vi "AlliGator Action Loop.vi"(8 "Error In":errorcluster, 10 "AlliGator Ctrl Refnums":T1, 11 "AlliGator Refnum":refnum<vi>) -> (0 "Error Out":errorcluster)   [LabVIEW 2021, in "AlliGator Action Engine.lvlib"]
doc: "AlliGator action dispatcher.\nEach action array is handled as a package, each action in the array being sent to the appropriate category (Files, Image, Phasor Graph, etc.)."
uses:
  AlliGator Action Engine.lvlib
  AlliGator Ctrl Refnums.ctl
  AlliGator Other Ctrl Refnums.ctl
  AlliGator State Indicator.ctl
  AlliGator Main Window Tabs.ctl
  AlliGator Phasor Plot Ctrl Refnums.ctl
  AlliGator Phasor Graph Ctrl Refnums.ctl
  Phasor/Phasor Calibration Type.ctl
  AlliGator Dataset Ctrl Refnums.ctl
  AlliGator Displayed Image.ctl
  AlliGator Registered Events Ctrl Refnums.ctl
  AlliGator Image Histogram Control Refnums.ctl
  Histograms/Linear Histogram Options.ctl
  Histograms/Histogram Bin Option.ctl
  Histograms/Histogram Bin Position.ctl
  AlliGator Decay Fit Map Control Refnums.ctl
  Fits/IRF(X)PSED/Decay Fit Parameters & Derived Quantities List.ctl
  AlliGator Internal Variables v2.ctl
  <vilib>/vision/Image Controls.llb/IMAQ Image.ctl
  AlliGator Gate Image Set.ctl
  AlliGator FLI Dataset Type.ctl
  AlliGator Data Series Type.ctl
  AlliGator Dataset Channel.ctl
  AlliGator Gate Arithmetic.ctl
  Image/Named ROI Description.ctl
  AlliGator Decay Metadata v3.ctl
  AlliGator Decay Background Subtraction Info.ctl
  AlliGator Baseline Subtraction Method.ctl
  Graphs/XY Graph/XY Graph Plot Shift Parameters.ctl
  Graphs/XY Graph/XY Graph Plot Shift Method.ctl
  AlliGator Decay Extrapolation Parameters.ctl
  Phasor/Calibration Phasor (m, phi).ctl
  Phasor/Phasor Reference Series.ctl
  Phasor/Phasor Calibration Map v2.ctl
  Phasor/Phasor (g, s).ctl
  AlliGator Raw Phasor Plot Data v4.ctl
  Phasor/Phasor Standard Deviation Options.ctl
  AlliGator Phasor Multi-Harmonic Data.ctl
  Phasor/Phasor Harmonic Data.ctl
  AlliGator Decay Fit Options & Parameters v2.ctl
  Fits/IRF(X)PSED/Decay Fit Options v2.ctl
  Fits/Decay Convolution/Decay Model.ctl
  Fits/Residual Type.ctl
  Fits/IRF(X)PSED/Fit Weights Type.ctl
  Fits/Non-linear Fitting Method v2.ctl
  Fits/Fit Calculation Method.ctl
  Fits/Non-linear Fitting Algorithm.ctl
  AlliGator Decay Fit Parameter Constraints 2.ctl
  Fits/IRF(X)PSED/Decay Fit Parameters In List.ctl
  Fits/IRF(X)PSED/MLE Baseline Offset Type.ctl
  AlliGator Decay Preprocessing Parameters.ctl
  AlliGator Parameter Maps Data.ctl
  AlliGator Q Event.ctl
  AlliGator Settings List.ctl
  Graphs/XY Graph/XY Graph Selected Plot Info.ctl
  Graphs/XY Graph/XY Graph Refnum.ctl
  <vilib>/Utility/miscctls.llb/LVPoint32TypeDef.ctl
  Graphs/XY Graph/XY Graph Mouse Click Event Data.ctl
  AlliGator Debug Action List.ctl
  Alligator Elements Order in Action Stack.ctl
  bb653f8f-7323-4417-bc10-ef5a2241dee5.vi
  AlliGator Globals.vi
  Variant/Variant to Data/Variant to Boolean.vi
  AlliGator Add Action Array to Stack.vi
  Error/Error.lvlib
  Utilities/Utilities.lvlib
  AlliGator GUI.lvlib
  Notebook/Notebook.lvlib
  AlliGator Globals, Variables & Constants.lvlib
  AlliGator Settings.lvlib
  Graphs/XY Graph/XY Graph Add-Ons.lvlib
  Variant/Variant to Data/Variant to Data.lvlib
  AlliGator Debug.lvlib
  Phasor/Phasor.lvlib
  Image/Image.lvlib
  AlliGator Decay Preprocessing.lvlib
  AlliGator Phasor Graph.lvlib
  AlliGator Files.lvlib
  AlliGator Internal Variables.lvlib
  AlliGator Phasor Plot.lvlib
  AlliGator Source Image.lvlib
  Fits/Fits.lvlib
  AlliGator Decay Fit.lvlib
  AlliGator Decay Fit Parameter Map.lvlib
  AlliGator Python Plugins.lvlib
  AlliGator Dual-Channel Datasets.lvlib
  Histograms/Histogram Window.lvlib
panel:
  # "Drop the content of this VI on AlliGator's diagram\nIn AlliGator, replace the subVI template by a new version"
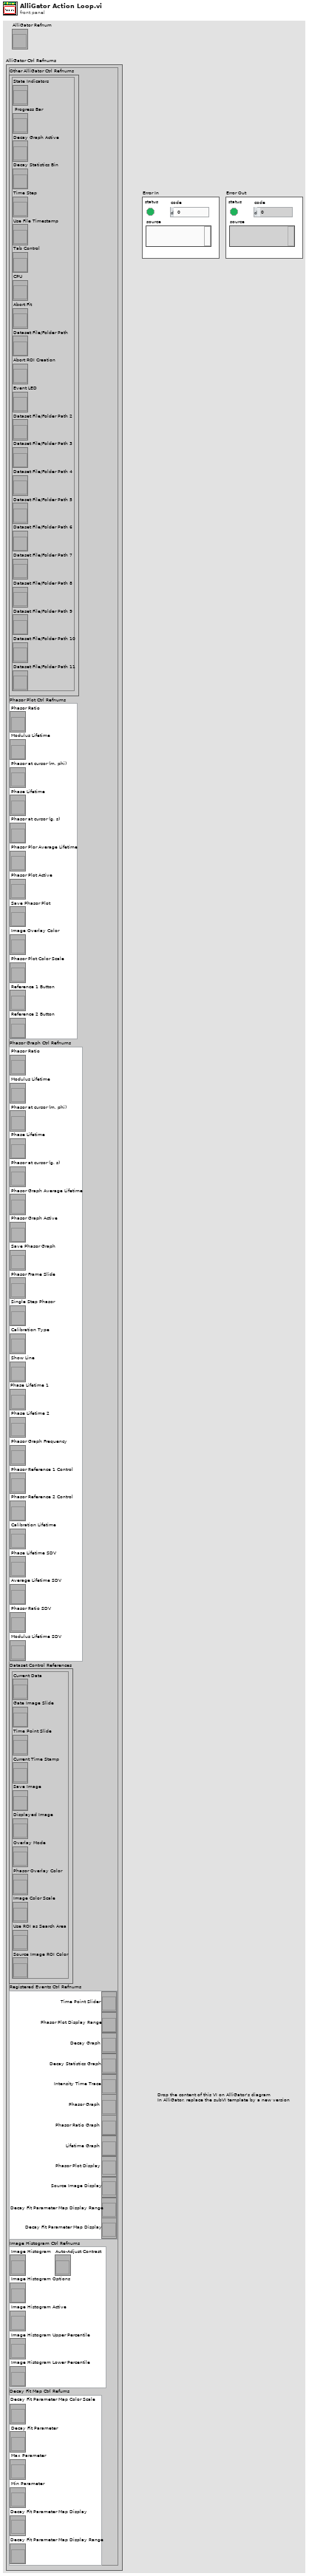
[diagram p1: front panel]
types:
  T1 = typedef "AlliGator GUI.lvlib/AlliGator Ctrl Refnums.ctl" = cluster{"Other AlliGator Ctrl Refnums":T2, "Phasor Plot Ctrl Refnums":T3, "Phasor Graph Ctrl Refnums":T4, "Dataset Control References":T5, "Registered Events Ctrl Refnums":T6, "Image Histogram Ctrl Refnums":T7, "Decay Fit Map Ctrl Refums":T8}
  T2 = typedef "AlliGator GUI.lvlib/AlliGator Other Ctrl Refnums.ctl" = cluster{"State Indicators":refnum<vi>, " Progress Bar":refnum<vi>, "Decay Graph Active":refnum<vi>, "Decay Statistics Bin":refnum<vi>, "Time Step":refnum<vi>, "Use File Timestamp":refnum<vi>, "Tab Control":refnum<vi>, "CPU":refnum<vi>, "Abort Fit":refnum<vi>, "Dataset File/Folder Path":refnum<vi>, "Abort ROI Creation":refnum<vi>, "Event LED":refnum<vi>, "Dataset File/Folder Path 2":refnum<vi>, "Dataset File/Folder Path 3":refnum<vi>, "Dataset File/Folder Path 4":refnum<vi>, "Dataset File/Folder Path 5":refnum<vi>, "Dataset File/Folder Path 6":refnum<vi>, "Dataset File/Folder Path 7":refnum<vi>, "Dataset File/Folder Path 8":refnum<vi>, "Dataset File/Folder Path 9":refnum<vi>, "Dataset File/Folder Path 10":refnum<vi>, "Dataset File/Folder Path 11":refnum<vi>}
  T3 = typedef "AlliGator GUI.lvlib/AlliGator Phasor Plot Ctrl Refnums.ctl" = cluster{"Phasor Ratio":refnum<vi>, "Modulus Lifetime":refnum<vi>, "Phasor at cursor (m, phi)":refnum<vi>, "Phase Lifetime":refnum<vi>, "Phasor at cursor (g, s)":refnum<vi>, "Phasor Plor Average Lifetime":refnum<vi>, "Phasor Plot Active":refnum<vi>, "Save Phasor Plot":refnum<vi>, "Image Overlay Color":refnum<vi>, "Phasor Plot Color Scale":refnum<vi>, "Reference 1 Button":refnum<vi>, "Reference 2 Button":refnum<vi>}
  T4 = typedef "AlliGator GUI.lvlib/AlliGator Phasor Graph Ctrl Refnums.ctl" = cluster{"Phasor Ratio":refnum<vi>, "Modulus Lifetime":refnum<vi>, "Phasor at cursor (m, phi)":refnum<vi>, "Phase Lifetime":refnum<vi>, "Phasor at cursor (g, s)":refnum<vi>, "Phasor Graph Average Lifetime":refnum<vi>, "Phasor Graph Active":refnum<vi>, "Save Phasor Graph":refnum<vi>, "Phasor Frame Slide":refnum<vi>, "Single Step Phasor":refnum<vi>, "Calibration Type":refnum<vi>, "Show Line":refnum<vi>, "Phase Lifetime 1":refnum<vi>, "Phase Lifetime 2":refnum<vi>, "Phasor Graph Frequency":refnum<vi>, "Phasor Reference 1 Control":refnum<vi>, "Phasor Reference 2 Control":refnum<vi>, "Calibration Lifetime":refnum<vi>, "Phase Lifetime SDV":refnum<vi>, "Average Lifetime SDV":refnum<vi>, "Phasor Ratio SDV":refnum<vi>, "Modulus Lifetime SDV":refnum<vi>}
  T5 = typedef "AlliGator GUI.lvlib/AlliGator Dataset Ctrl Refnums.ctl" = cluster{"Current Data":refnum<vi>, "Gate Image Slide":refnum<vi>, "Time Point Slide":refnum<vi>, "Current Time Stamp":refnum<vi>, "Save Image":refnum<vi>, "Displayed Image":refnum<vi>, "Overlay Mode":refnum<vi>, "Phasor Overlay Color":refnum<vi>, "Image Color Scale":refnum<vi>, "Use ROI as Search Area":refnum<vi>, "Source Image ROI Color":refnum<vi>}
  T6 = typedef "AlliGator GUI.lvlib/AlliGator Registered Events Ctrl Refnums.ctl" = cluster{"Time Point Slider":refnum<vi>, "Phasor Plot Display Range":refnum<vi>, "Decay Graph":refnum<vi>, "Decay Statistics Graph":refnum<vi>, "Intensity Time Trace":refnum<vi>, "Phasor Graph":refnum<vi>, "Phasor Ratio Graph":refnum<vi>, "Lifetime Graph":refnum<vi>, "Phasor Plot Display":refnum<vi>, "Source Image Display":refnum<vi>, "Decay Fit Parameter Map Display Range":refnum<vi>, "Decay Fit Parameter Map Display":refnum<vi>}
  T7 = typedef "AlliGator GUI.lvlib/AlliGator Image Histogram Control Refnums.ctl" = cluster{"Image Histogram":refnum<vi>, "Image Histogram Options":refnum<vi>, "Image Histogram Active":refnum<vi>, "Image Histogram Upper Percentile":refnum<vi>, "Image Histogram Lower Percentile":refnum<vi>, "Auto-Adjust Contrast":refnum<vi>}
  T8 = typedef "AlliGator Decay Fit Parameter Map.lvlib/AlliGator Decay Fit Map Control Refnums.ctl" = cluster{"Decay Fit Parameter Map Color Scale":refnum<vi>, "Decay Fit Parameter":refnum<vi>, "Max Parameter":refnum<vi>, "Min Parameter":refnum<vi>, "Decay Fit Parameter Map Display":refnum<vi>, "Decay Fit Parameter Map Display Range":refnum<vi>}
  T9 = typedef "AlliGator Internal Variables.lvlib/AlliGator Internal Variables v2.ctl" = cluster{"Displayed Image":T10, "White Light Image":T10, "Mask Image":T10, "ROI Mask Image":T10, "Current Dataset Images 1":T11, "Background Dataset Images 1":T11, "Current Dataset Images 2":T11, "Background Dataset Images 2":T11, "Current Dataset Arithmetic Images":T11, "Accumulated Dataset Images 1":T11, "Accumulated Dataset Images 2":T11, "Accumulated Dataset Arithmetic Images":T11, "Phasor Plot Image":T10, "Decay Fit Parameter Map Image":T10, "Single Data Point Path":path, "White Light Image Path":path, "Mask Image Path":path, "Time-Series Folder":path, "[Time-Series Paths]":path[], "Current Dataset":i32, "Single Dataset Type":T12, "Current Folder":string, "AlliGator Data Series Type":T13, "# Datasets":i32, "Dual-Channel Dataset":bool, "Selected Channel Name":string, "Dataset Channel":T14, "Channel Arithmetic":T15, "Dual-Channel Background Dataset":bool, "Background Channel":T14, "Dual-Channel Accumulated Dataset":bool, "Start Time":dbl, "[Time-Series Timestamps]":dbl[], "[Intensity Corrections]":dbl[], "Time Series Script":bool, "Type of Displayed Image":T16, "Gate Image Slide":u16, "# Gates":i32, "ROIs":T17[], "ROI Decay":cluster{"t Array":dbl[], "I Array":dbl[]}, "Valid Decay":bool, "Decay  Metadata":T19, "Reference Decay Plot Name":string, "Reference Decay":cluster{"t Array":dbl[], "I Array":dbl[]}, "Decay Shift Plot":cluster{"Time Stamps":dbl[], "Decay Shifts":dbl[]}, "[Decays Max Values]":sgl[], "[Decays Min Values]":sgl[], "Calibration Phasor":T25, "Calibration Phasor Series":T26, "Phasor Calibration Map":T27, "Calibration Map MD5 Digest":string, "Last Raw Phasor":T28, "Last Calibrated Phasor":T28, "Last Calibrated Phasor SDV":T28, "Phasor Graph:Phasor Plot":cluster{"g Array":dbl[], "s Array":dbl[]}, "Phasor Graph:Phasor SDV Plot":cluster{"g Array":dbl[], "s Array":dbl[]}, "[Phasor Graph:Raw Phasor Plots]":T29[], "Phasor Plot locked to Ref 1":i32, "[Phasor Plot(s) locked to Ref 1]":i32[], "[Phasor Plot(s) locked to Ref 2]":i32[], "[Pixel Phasors]":T28[], "[[Sum Image]]":dbl[][], "[[CSG Phasors]]":csg[][], "[[Valid Pixel?]]":bool[][], "I/m/phi Dataset":cluster{"I/m/phi Dataset?":bool, "Base Frequency":dbl[unit], "Harmonic Orders":u8[]}, "Multi Phasor Plot Data":T31, "Decay Fit Options & Parameters":T33, "Fit Options: Decay Preprocessing Parameters":T44, "Fit Options: Reference Decay":cluster{"t Array":dbl[], "I Array":dbl[]}, "Is Full Image Parameters Map":bool, "Is Single-Pixels Parameters Map":bool, "NLSF Parameters Map X Resolution":i32, "NLSF Parameters Map Y Resolution":i32, "[Single Decay Fit Parameters]":dbl[], "Fit Model":T35, "[[Multiple Decays Fit Parameters]]":dbl[][], "[[Multiple Decays Fit Parameter SDVs]]":dbl[][], "[[IRFs]]":dbl[][], "IRF Array Time Axis":dbl[], "Decay Array Time Axis":dbl[], "[Decay Fit Parameter Names]":T45[], "[[Phasor Ratios]]":dbl[][], "[[Average Lifetimes]]":dbl[][], "Amplitude Weighted Average Lifetime":bool, "[Decay Sum]":dbl[], "Parameter Maps":T46[], "[[User-defined Quantities]]":dbl[][], "User-defined Quantity":string}
  T10 = typedef "IMAQ Image.ctl" = refnum<image>
  T11 = typedef "AlliGator Internal Variables.lvlib/AlliGator Gate Image Set.ctl" = cluster{"SGL Image Max":T10, "SGL Image Sum":T10, "SGL Gate Images":T10[], "SGL Image Min":T10}
  T12 = typedef "AlliGator Files.lvlib/AlliGator FLI Dataset Type.ctl" = enum16{"HDF5 FLI Dataset", "Gate Image Folder", ".sdt FLI Dataset (Becker & Hickl)", ".ptu FLI Dataset (PicoQuant)", "SS1 FLI Dataset", "SS2 FLI Dataset", "I/m/phi Dataset", ".bin FLI Dataset (PicoQuant Binned)", ".bin FLI Dataset (Piccolo Binned)"}
  T13 = typedef "AlliGator Files.lvlib/AlliGator Data Series Type.ctl" = enum16{"Not a Supported Series", "Gate Images Folder Series", "SwissSPAD 2 Dataset Series", "B&H FLI Dataset Series", "PicoQuant PTU FLI Dataset Series", "PicoQuant BIN FLI Dataset Series", "Piccolo hist BIN FLI Dataset Series", "HDF5 FLI Dataset Series"}
  T14 = typedef "AlliGator Dual-Channel Datasets.lvlib/AlliGator Dataset Channel.ctl" = enum16{"G2", "INT"}
  T15 = typedef "AlliGator Settings.lvlib/AlliGator Gate Arithmetic.ctl" = enum16{"None", "INT-G2", "G2/INT*<INT>", "(1 - G2/INT)*<INT>"}
  T16 = typedef "AlliGator Source Image.lvlib/AlliGator Displayed Image.ctl" = enum16{"Single Gate", "Sum of All Gates", "Max of All Gates", "Min of All Gates", "-", "White Ligth Image", "Mask Image"}
  T17 = typedef "Image.lvlib/Named ROI Description.ctl" = cluster{"ROI Descriptor":T18, "ROI Name":string, "Overlay Color":u32}
  T18 = typedef "ROI Descriptor" = cluster{"Global Rectangle":i32[], "Contours":cluster{"ID":enum32{"External", "Internal"}, "Type":u32, "Coordinates":i32[]}[]}
  T19 = typedef "AlliGator Phasor Graph.lvlib/AlliGator Decay Metadata v3.ctl" = cluster{"ROI Descriptor":T18, "ROI Center":cluster{"X":i32, "Y":i32}, "Decay Background Subtraction Info":T20, "Decay Reverted":bool, "Decay Smoothened":bool, "Decay Straightened":bool, "Fitted Tau (Decay Straightening)":dbl, "Decay Shift Parameters":T22, "Decay Shifted":bool, "Decay Extrapolated":bool, "Decay Extrapolation Parameters":T24, "Decay Normalized":bool, "Fold Decay":bool, "# Folds":u32}
  T20 = typedef "AlliGator Decay Analysis.lvlib/AlliGator Decay Preprocessing.lvlib/AlliGator Decay Background Subtraction Info.ctl" = cluster{"Laser Period":dbl[unit], "Gate Duration":dbl[unit], "Baseline Subtraction Method":T21, "Background Definition Range":cluster{"Min Gate":dbl[unit], "Max Gate":dbl[unit]}, "Total Intensity w/o Bkgd Subtraction":dbl, "Bkgd-subtracted Intensity (exp)":dbl, "# Data Points":i32, "Background/Gate":dbl, "Fitted Lifetime":dbl[unit], "Bkgd-subtracted Intensity (theo)":dbl}
  T21 = typedef "AlliGator Decay Analysis.lvlib/AlliGator Decay Preprocessing.lvlib/AlliGator Baseline Subtraction Method.ctl" = enum16{"Mean", "Min", "Square Gated Single-Exponential", "File", "Constant"}
  T22 = typedef "XY Graph Add-Ons.lvlib/XY Graph Plot Shift Parameters.ctl" = cluster{"Type":T23, "Shift":dbl[unit], "Threshold":dbl, "Rotate":bool}
  T23 = typedef "XY Graph Add-Ons.lvlib/XY Graph Plot Shift Method.ctl" = enum16{"Default", "CFD", "Threshold", "Cross-Correlation"}
  T24 = typedef "AlliGator Decay Analysis.lvlib/AlliGator Decay Preprocessing.lvlib/AlliGator Decay Extrapolation Parameters.ctl" = cluster{"Additional Points":u32, "Head Fraction":dbl, "Fitted Tau":dbl, "Use Periodicity":bool, "Use Cursors":bool, "Tail Fraction":dbl}
  T25 = typedef "Phasor.lvlib/Calibration Phasor (m, phi).ctl" = cluster{"m":dbl, "phi":dbl, "Phasor Frequency":dbl[unit], "Reference Lifetime":dbl[unit]}
  T26 = typedef "Phasor.lvlib/Phasor Reference Series.ctl" = cluster{"m Array":dbl[], "phi Array":dbl[], "Phasor Frequency":dbl[unit], "Calibration Lifetime":dbl[unit]}
  T27 = typedef "Phasor.lvlib/Phasor Calibration Map v2.ctl" = cluster{"Phasor Frequency":dbl[unit], "Calibration Lifetime":dbl[unit], "ROI Centers":cluster{"X":i32, "Y":i32}[], "ROI Descriptors":T18[], "Map Resolution X":i32, "Map Resolution Y":i32, "z Array":cdb[]}
  T28 = typedef "Phasor.lvlib/Phasor (g, s).ctl" = cluster{"g":dbl, "s":dbl}
  T29 = typedef "AlliGator Phasor Graph.lvlib/AlliGator Raw Phasor Plot Data v4.ctl" = cluster{"Phasor Plot Name":string, "Raw Phasor Plot":T28[], "Phasor Frequency":dbl[unit], "[Decay Metadata]":T19[], "Raw Phasor Plot SDV":T28[], "Phasor SDV Options":T30, "[Calibration Phasor]":T25[]}
  T30 = typedef "Phasor.lvlib/Phasor Standard Deviation Options.ctl" = cluster{"Compute Estimated SDV":bool, "# Replicas":u32, "Use Estimated Average Phasor":bool}
  T31 = typedef "AlliGator Phasor Plot.lvlib/AlliGator Phasor Multi-Harmonic Data.ctl" = cluster{"Base Frequency":dbl[unit], "# Harmonics":u8, "Harmonic Orders":u8[], "Phasor Plot Settings Checksum":u64, "Phasor Harmonic Data Array":T32[]}
  T32 = typedef "Phasor.lvlib/Phasor Harmonic Data.ctl" = cluster{"Phasor Harmonic Name":string, "Phasor Plot Settings Checksum":u64, "Phasor Frequency":dbl[unit], "Base Frequency":dbl[unit], "Harmonic Order":u8, "Phasor Plot Parameters":string, "Phasor Array [[CSG]]":csg[][], "Dataset File Path":path}
  T33 = typedef "AlliGator Decay Fit Parameter Map.lvlib/AlliGator Decay Fit Options & Parameters v2.ctl" = cluster{"SYNC Period":dbl[unit], "Fit Options":T34, "Fit Parameter Constraints":T41[], "MLE Baseline Offset":dbl, "MLE Baseline Offset Type":T43}
  T34 = typedef "Fits.lvlib/Decay Fit Options v2.ctl" = cluster{"Show Fit Residuals":bool, "Fit Model":T35, "Residual Type":T36, "Max Decay Percentile":dbl, "Min Decay Percentile":dbl, "Show Full Decay":bool, "Weights":T37, "Fitting Method":T38, "Compute Parameter Uncertainties":bool, "Periodic Boundaries":bool, "Model Calculation":T39, "Period":dbl[unit], "Termination Criteria":cluster{"Max Iterations":i32, "Max Function Calls":i32, "Max Time":dbl[unit], "Function Tolerance":dbl, "Parameter Tolerance":dbl, "Gradient Tolerance":dbl, "Min Lambda":dbl, "Max Lambda":dbl, "Initial Tick Count":u32}, "Offset Resolution":dbl[unit], "Use Local IRF":bool, "Fitting Algorithm":T40}
  T35 = typedef "Fits.lvlib/Decay Model.ctl" = enum16{"1-Exponential", "2-Exponentials"}
  T36 = typedef "Fits.lvlib/Residual Type.ctl" = enum16{"Standard", "Normalized", "Reduced"}
  T37 = typedef "Fits.lvlib/Fit Weights Type.ctl" = enum16{"Unweighted", "1/Variance", "Best of All"}
  T38 = typedef "Fits.lvlib/Non-linear Fitting Method v2.ctl" = enum16{"Least Square", "Least Absolute Residual", "Bisquare", "MLE", "-", "Best of All"}
  T39 = typedef "Fits.lvlib/Fit Calculation Method.ctl" = enum16{"Simulation", "Convolution", "Integration"}
  T40 = typedef "Fits.lvlib/Non-linear Fitting Algorithm.ctl" = enum16{"Levenberg-Marquardt", "Trust-Region Dogleg"}
  T41 = typedef "AlliGator Decay Analysis.lvlib/AlliGator Decay Fit.lvlib/AlliGator Decay Fit Parameter Constraints 2.ctl" = cluster{"Fit Parameter":T42, "Min Value":dbl, "Max Value":dbl, "Global":bool, "Used":bool}
  T42 = typedef "Fits.lvlib/Decay Fit Parameters In List.ctl" = enum16{"Offset", "Baseline", "A_1", "tau_1", "A_2", "tau_2"}
  T43 = typedef "Fits.lvlib/MLE Baseline Offset Type.ctl" = enum32{"Absolute", "Percentage"}
  T44 = typedef "AlliGator Decay Analysis.lvlib/AlliGator Decay Preprocessing.lvlib/AlliGator Decay Preprocessing Parameters.ctl" = cluster{"Background Subtraction":bool, "Straighten Decay":bool, "Reverse Gates":bool, "1-Normalized Decay":bool, "Smoothen Decay":bool, "Smoothing Parameter":dbl, "Shift Decay":bool, "Decay Shift Parameters":T22, "Extrapolate Decay":bool, "Additional Points":u32, "Head Fraction":dbl, "Pixel-Normalize Decay":bool, "Use Periodicity":bool, "Use Cursors":bool, "Tail Fraction":dbl, "Use Decay Pre-Processing":bool, "Fold Decay":bool, "# Folds":u32, "[0-1]-Normalized Decay":bool}
  T45 = typedef "Fits.lvlib/Decay Fit Parameters & Derived Quantities List.ctl" = enum16{"Offset", "Baseline", "A_1", "tau_1", "A_2", "tau_2", "<tau>_a", "f1_a", "f2_a", "<tau>_i", "f1_i", "f2_i", "-", "R^2", "Chi^2"}
  T46 = typedef "AlliGator Parameter Maps Data.ctl" = cluster{"Map Set Name":string, "[Parameter Names]":string[], "[[Parameters]]":dbl[][], "[[Parameter SDVs]]":dbl[][], "Decay Array Time Axis":dbl[], "[[IRFs]]":dbl[][], "IRF Array Time Axis":dbl[]}
  T47 = typedef "AlliGator Action Engine.lvlib/AlliGator Q Event.ctl" = enum16{"---- Files ----", "Files:Set Batch Export Files To Save", "Files:Set Dataset Loading & Pre-processing Options", "Files:Check #Frames in Dataset", "Files:Increment Frame Index", "Files:Open Mask Image", "Files:Open White Light Image", "Files:Open Single Dataset", "Files:New Folder of Folders Selected", "Files:Load File (all Types)_Scriptable", "Files:Move Flattened Series to Folders Series", "Files:Select Folder", "Files:Load FLI Dataset", "Files:Load Swiss SPAD 1 Dataset", "Files:Load Swiss SPAD 2 Dataset", "Files:Load .sdt FLI Dataset", "Files:Load .ptu FLI Dataset", "Files:Load .bin FLI Dataset", "Files:Load Single Gate Image Folder", "Files:Load I/m/phi Dataset (deprecated)", "Files:Load Single Image", "Files:Subtract Background File", "Files:Export FLI Dataset", "Files:Load HDF5 FLI Dataset", "Files:Set Destination File Path", "Files:Save Mask Image", "Files:Batch Conversion", "Files:New Folder Selected", "Files:Close FLI Dataset", "Files:Close FLI Dataset Series", "Files:Close White Light Image", "Files:Close Mask Image", "---- FLI Dataset ----", "FLI Dataset:Channel Arithmetic", "FLI Dataset:Export Average Lifetime Map as ASCII", "FLI Dataset:Export User-Defined Quantity Map as ASCII", "FLI Dataset:Python Function FLI Dataset Event", "FLI Dataset:ROI Analysis", "FLI Dataset:Tilted Logistic Square Gated IRF Characteristics Map", "FLI Dataset:Logistic Square Gated IRF Characteristics Map", "FLI Dataset:Square Gated IRF Characteristics Map", "FLI Dataset:Multi-ROI Single-Pixel Phasor Analysis", "FLI Dataset:Multi-ROI Single-Pixel NLSF Analysis", "FLI Dataset:All ROIs IRF Extraction", "FLI Dataset:All ROIs Decay Fit Non-Interactive (Fast + Individual IRF)", "FLI Dataset:All ROIs Phasor Analysis", "FLI Dataset:All ROIs Decay Fit", "FLI Dataset:Fluorescence Decay Statistics", "FLI Dataset:Update Decay Statistics Graph", "FLI Dataset:Get Decay from ROI", "FLI Dataset:All ROIs Average Lifetimes", "---- FLI Dataset Series ----", "FLI Dataset Series:Sum All Datasets in Series", "FLI Dataset Series:Add Dataset to Accumulated Dataset", "FLI Dataset Series:Display Accumulated Dataset", "FLI Dataset Series:Clear Dataset Series Sum", "FLI Dataset Series:Time-Series Analysis (NLSF)", "FLI Dataset Series:Time-Series Analysis (Phasor)", "---- Image ----", "Image:Update Image Profile Plots", "Image:Image Histogram Cursor Move", "Image:Image Histogram", "Image:Image Contrast", "Image:Set Image Histogram Cursor Move Flag", "Image:Clear Image Overlay", "Image:Use ROI as Search Area", "Image:Set ROI Diameter", "Image:Save Image Data as TIFF", "Image:Save Displayed Image with Overlay", "Image:Save Image Overlay Only", "Image:Save Image as Hot Pixel Mask", "Image:Change Source Image Color Palette", "Image:Copy Image to Clipboard", "Image:Source Image ROI Selection", "Image:Delete All ROIs", "Image:Delete All Unselected ROIs", "Image:Delete ROI", "Image:Merge All ROIs", "Image:Store ROI", "Image:Source Image ROI Storage", "Image:Export ROI Description to Notebook", "Image:Save ROI", "Image:Load ROI", "Image:Paste ROI Definition", "Image:Clear ROI", "Image:Identify ROIs in Mask Image", "Image:Create Complementary ROI", "Image:Create Contour ROI", "Image:Create ROI(s) from Pixels with Peak above Min_Scriptable", "Image:Create ROI(s) from Pixels with Intensity above Min_Scriptable", "Image:Compute ROI Statistics", "Image:Delete ROI(s) based on ROI Characteristics", "Image:Create ROI Grid", "Image:ROI to Individual Pixel ROIs", "Image:Python Function Source Image Event", "Image:Show Phasor Calibration Map ROI Centers", "Image:Convert ROI to Mask Image", "Image:Mouse Move", "Image:Mouse Up", "Image:Set Source Image Mouse Move Flag", "Image:Add Scale Bar Overlay", "Image:Delete Existing ROIs Option", "Image:Overlay ROI Median", "---- Decay ----", "Decay:Clear IRF/Reference Plot", "Decay:Clear Local IRFs", "Decay:Add Decay to Graph", "Decay:Smoothen Plot", "Decay:Smoothen Plot Tail", "Decay:Average Selected Plots", "Decay:Extract IRF", "Decay:Optimal IRF Extraction", "Decay:Threshold IRF", "Decay:Fit to Model IRF", "Decay:Fit IRF to Square Gate", "Decay:Fit IRF to Logistic Square Gate", "Decay:Fit IRF to Tilted Logistic Square Gate", "Decay:Create Bounding Cursors Set", "Decay:Export Bounding Cursors Definition to Notebook", "Decay:Denoise Plot", "Decay:Compute Cumulative Function", "Decay:Use as Reference Decay", "Decay:Show Reference Decay/IRF", "Decay:Extrapolate Decay", "Decay:Create Head & Tail Bounding Cursors", "Decay:Store Cursor-defined Head & Tail Fractions", "Decay:Rebin Plot", "Decay:1-Normalize Decay", "Decay:[0-1]-Normalize Plot", "Decay:Straighten Decay", "Decay:Shift Decay", "Decay:Fold Decay", "Decay:Fit Decay", "Decay:Global Fit of Selected Decays", "Decay:Post Global Fit Script", "Decay:Add Global Fit Parameters to Graph", "Decay:Add Decay Parameter(s) to Plot (Graph)", "Decay:Export Decay to Phasor Graph", "Decay:Plot Decay Shifts", "Decay:Compute Average Lifetime", "Decay:Plot Convolution", "Decay:Graph Tip Strip Update", "---- Decay Statistics ----", "Decay Statistics:Tip Strip Update", "---- Intensity Time Trace ----", "Intensity Time Trace:Use File Timestamp", "Intensity Time Trace:Load Intensity Corrections File", "Intensity Time Trace:Clear Intensity Corrections File", "Intensity Time Trace:Tip Strip Update", "---- Phasor Plot ----", "Phasor Plot:Build Phasor Plot", "Phasor Plot:Change Phasor Plot Color Palette", "Phasor Plot:Adjust Phasor Plot Display Range", "Phasor Plot:Highlight Image ROI in Phasor Plot", "Phasor Plot:Save Phasor Plot Image with Overlay", "Phasor Plot:Export Complex Phasor Map", "Phasor Plot:Export Phasor Ratio Map", "Phasor Plot:Export Average Lifetime Map", "Phasor Plot:Compute Phase Lifetime Histogram", "Phasor Plot:Compute Phasor Ratio Histogram", "Phasor Plot:Compute Phase Lifetime vs Intensity Scatter Plot", "Phasor Plot:Weber 2-Component Decomposition", "Phasor Plot:Update Phasor Color Map Vertices", "Phasor Plot:Clear Phasor Overlay", "Phasor Plot:Use Segment Extremities as References", "Phasor Plot:Use UC/Segment Intersections as References", "Phasor Plot:Use UC/Principal Axis Intersections as References", "Phasor Plot:Use UC/Linear Fit Intersections as References", "Phasor Plot:Update Phasor Plot Reference", "Phasor Plot:Show Local Phasor Info in Phasor Plot", "Phasor Plot:Update Phasor Plot State", "Phasor Plot:Phasor Plot ROI Storage", "Phasor Plot:Phasor Plot ROI Selection", "Phasor Plot:Python Function Phasor Plot Event", "Phasor Plot:Overlay Phasor ROI, Ratio or Map in Source Image", "Phasor Plot:Compute Decay of Selected Phasors", "Phasor Plot:Phasor at Image Pixel", "Phasor Plot:Mouse Move", "Phasor Plot:Mouse Up", "Phasor Plot:Display Range Mouse Move", "Phasor Plot:Set Mouse Move Flag", "---- Phasor Graph ----", "Phasor Graph:Calibrated Phasor Map Series", "Phasor Graph:Whole Image Phasor Scatter Plot (Todo)", "Phasor Graph:Get Phasor Value", "Phasor Graph:Create New Phasor Plot Dialog", "Phasor Graph:Update Last Phasor Value", "Phasor Graph:Update Phasor (m, phi)", "Phasor Graph:Remove Single Phasor from Plot", "Phasor Graph:Add Single Phasor to Plot", "Phasor Graph:Remove Phasor Plot", "Phasor Graph:Remove Selected Phasor Plots", "Phasor Graph:Clear Phasor Data", "Phasor Graph:Clear Phasor Graph", "Phasor Graph:Cursor Move", "Phasor Graph:Draw Cursor Connecting Line", "Phasor Graph:Clear Cursor Connecting Line", "Phasor Graph:Find UC Intersection", "Phasor Graph:Use UC/Cursor-Defined Line Intersections", "Phasor Graph:Use Selected Plots Fitted Line/UC Intersections", "Phasor Graph:Use Selected Plots Principal Axis/UC Intersections", "Phasor Graph:Show Single Phasor", "Phasor Graph:Save Single Phasor Plot", "Phasor Graph:Save All Phasor Plots", "Phasor Graph:Load Phasor Plot(s)", "Phasor Graph:Phasor Multiplication", "Phasor Graph:Compute Average Phasor", "Phasor Graph:Compute Multiple Average Phasors (Selected Plots)", "Phasor Graph:Export Single Phasor Plot Phase Lifetimes", "Phasor Graph:Phase Lifetime Trajectory", "Phasor Graph:Phase Lifetime vs Intensity Scatter Plot (deprecated)", "Phasor Graph:Parameter 2 vs Parameter 1 Scatter Plot", "Phasor Graph:Use Cursor n Location", "Phasor Graph:Set Reference n to Current Phase Lifetime Value", "Phasor Graph:Set Reference n to Lifetime Value", "Phasor Graph:Set Cursor n Location", "Phasor Graph:Save Phasor Graph Image", "Phasor Graph:Update SEPL Plot", "Phasor Graph:Export Single Phasor Plot Data", "Phasor Graph:Export Selected Phasor Plots Data", "Phasor Graph:Python Function Phasor Graph Event", "Phasor Graph:Tip Strip Update", "---- Calibration ----", "Calibration:Set Calibration Type", "Calibration:Load/Save Phasor Calibration", "Calibration:Load/Save Phasor Calibration Series", "Calibration:Load/Save Phasor Calibration Map", "Calibration:Use as Calibration", "Calibration:Compute Optimal Calibration from Phasor References", "Calibration:Clear Phasor Calibration", "Calibration:Single Phasor Calibration Information", "Calibration:Use as Calibration Series", "Calibration:Use as Calibration Map", "Calibration:Clear Calibration Series", "Calibration:Phasor Calibration Series Information", "Calibration:Clear Calibration Map", "Calibration:Phasor Calibration Map Information", "Calibration:Apply Phasor Calibration", "Calibration:Update Single Plot Calibration", "Calibration:Update Multiple Plots Calibration", "Calibration:Clear Single Plot Calibration", "Calibration:Clear All Plots Calibrations", "Calibration:Clear Plot(s) Calibration(s)?", "Calibration:Phasor Calibration Maps (# Gates Series)", "---- Phasor Ratio ----", "Phasor Ratio:Clear Reference n", "Phasor Ratio:Toggle Selected Plot(s)  Lock to Reference 1", "Phasor Ratio:Use as Reference n", "Phasor Ratio:Send Reference n to Notebook", "Phasor Ratio:Toggle Selected Plot(s)  Lock to Reference 2", "Phasor Ratio:Compute Phasor Ratio at Mouse Location", "Phasor Ratio:Compute Phasor Plot's Average Phasor Ratio", "Phasor Ratio:Compute Time-Series Phasor Ratios", "Phasor Ratio:Fit Line to Phasor Ratio Plot", "Phasor Ratio:Save References", "Phasor Ratio:Load References", "Phasor Ratio:Update Phasor Reference 1", "Phasor Ratio:Update Phasor Reference 2", "Phasor Ratio:Move Cursor n to Reference n", "Phasor Ratio:Use as Phasor Reference 1 Lifetime", "Phasor Ratio:Use as Phasor Reference 2 Lifetime", "Phasor Ratio:Export Phasor Ratio Map as ASCII", "Phasor Ratio:Tip Strip Update", "---- Lifetime & Other Parameters Graph ----", "Lifetime:Tip Strip Update", "---- Decay Fit Parameter Map ----", "Decay Fit Parameter Map:Export ROI NLSF Data as ASCII", "Decay Fit Parameter Map:Set Decay Fit  Parameter Map Selection", "Decay Fit Parameter Map:Build Decay Fit Parameter Map", "Decay Fit Parameter Map:Change Decay Fit Parameter Map Color Palette", "Decay Fit Parameter Map:Export Decay Fit Parameter Map Data as ASCII", "Decay Fit Parameter Map:Export All Decay Fit Parameter Maps Data as ASCII", "Decay Fit Parameter Map:Send Map Data to Lifetime Graph", "Decay Fit Parameter Map:Save Decay Fit Parameter Map Image", "Decay Fit Parameter Map:Save-Load IRFs & Fit Data", "Decay Fit Parameter Map:Update Local Decay Plots", "Decay Fit Parameter Map:Python Function Decay Fit Parameters Map Event", "Decay Fit Parameter Map:Overlay Decay Fit Parameter Map in Source Image", "Decay Fit Parameter Map:Plot Map Data vs Intensity", "Decay Fit Parameter Map:Mouse Up", "Decay Fit Parameter Map:Display Range Mouse Move", "---- Generic Graph ----", "Generic Graph:Generic XY Graph Event", "Generic Graph:Python Function XY Graph Event", "Generic Graph:New Plot", "Generic Graph:Save Plot", "Generic Graph:XY Plot Histogram", "Generic Graph:Set XY Graph Plot Name", "Generic Graph:Set Last Cursor Style", "Generic Graph:Tip Strip Update", "---- GUI ----", "GUI:Start Script", "GUI:Type of Displayed Image Changed", "GUI:Gate Image Slide Changed", "GUI:Show Busy Icon", "GUI:Show Busy Icon & Abort Button", "GUI:Hide Busy Icon", "GUI:Hide Busy Icon & Abort Button", "GUI:Abort", "GUI:End Script", "GUI:Start Timing", "GUI:End Timing", "GUI:Set State Indicator", "GUI:Send Parameters JSON Strings to Clipboard", "GUI:Set Gate Step", "GUI:Idle", "GUI:Initialization", "GUI:Quit", "GUI:Increment Dataset Index", "GUI:Set Dataset Index to -1", "GUI:Time Series Slider Moved", "GUI:Time Series Slider Changed", "GUI:Toggle Playback or Loop", "GUI:Playback Script", "GUI:Set Phasor Frequency", "GUI:Open Window", "GUI:Start Test Script", "GUI:End Test Script", "DEBUG"}
  T48 = typedef "XY Graph Add-Ons.lvlib/XY Graph Mouse Click Event Data.ctl" = cluster{"Multiplot XY Graph":T49, "Mouse Coordinates":T50}
  T49 = typedef "XY Graph Add-Ons.lvlib/XY Graph Refnum.ctl" = refnum<vi>
  T50 = typedef "LVPoint32TypeDef.ctl" = cluster{"Horizontal":i32, "Vertical":i32}
  T51 = typedef "XY Graph Add-Ons.lvlib/XY Graph Selected Plot Info.ctl" = cluster{"Multiplot XY Graph":T49, "Mouse Coordinates":T50, "Plot Index":i32}
  T52 = typedef "AlliGator Settings.lvlib/AlliGator Settings List.ctl" = enum16{"GUI:Visible Settings Tab", "GUI:Last Run Version", "Source Image:Use Image Histogram for Contrast", "Source Image:Low Count Pixels Rejection Options", "Source Image:High Count Pixels Rejection Options", "Source Image:Use Image Brightness", "Source Image:Blend Overlay with Image Background", "Source Image:Use Fixed ROI Diameter", "Source Image:ROI Diameter", "Source Image:ROI Center Color", "Source Image:Peak Threshold", "Source Image:Intensity Threshold", "Source Image:Image Binning Options", "Source Image:Image Smoothing Options", "Source Image:Image Histogram Active", "Source Image:Invert Binary Mask", "Source Image:Hot Pixel Removal", "Source Image:Overlay Analyzed ROI Center", "Source Image:Auto-Adjust Contrast", "Source Image:Histogram Lower Percentile", "Source Image:Histogram Upper Percentile", "Source Image:Save Source Image", "Source Image:Scale Bar Options", "Source Image:Image Resolution (Pixel Size)", "Source Image:Flatfield Correction", "Source Image:Show Dead Left Columns Correction", "Source Image:Dead Left Columns Correction", "Source Image:Image Pre-Processing Operations Order", "Source Image:Overlay ROI Median", "Source Image:Median Overlay Color", "Data Information:Gate Width", "Data Information:Nanotime Gate Separation", "Data Information:Macrotime Gate Separation", "Data Information:Gate Step", "Data Information:# Gates", "Data Information:Gate Image Exposure", "Data Information:Gate Image Integration", "Data Information:Gates to Skip", "Data Information:Gates to Keep", "Data Information:Define Gates to", "Data Information:Channel Name", "Data Information:Available Channel Names", "Data Information:Channel Arithmetic", "Data Information:Background File Subtraction", "Data Information:Background File", "Data Information:Background Scaling Factor", "Data Information:Background Pile-up Correction", "Data Information:Background Pixel Well Capacity", "Data Information:Laser Period", "Data Information:SYNC Period", "Data Information:Pile-up Correction", "Data Information:Pixel Well Capacity", "Data Information:Dataset Scaling Factor", "Fluorescence Decay_Decay Pre-Processing:Reverse Gates", "Fluorescence Decay_Decay Pre-Processing:Verbose Decay Pre-Processing", "Fluorescence Decay_Decay Pre-Processing:Use Decay Pre-Processing", "Fluorescence Decay_Decay Pre-Processing:Background Subtraction", "Fluorescence Decay_Decay Pre-Processing:Background Definition Range", "Fluorescence Decay_Decay Pre-Processing:Baseline Subtraction Method", "Fluorescence Decay_Decay Pre-Processing:Decay Pre-Processing Operations Order", "Fluorescence Decay_Decay Pre-Processing:Smoothing Parameter", "Fluorescence Decay_Decay Pre-Processing:Shift Decay", "Fluorescence Decay_Decay Pre-Processing:Decay Shift Parameters", "Fluorescence Decay_Decay Pre-Processing:Fold Decay", "Fluorescence Decay_Decay Pre-Processing:# Folds", "Fluorescence Decay_Decay Pre-Processing:1-Normalize Decay", "Fluorescence Decay_Decay Pre-Processing:[0-1]-Normalize Decay", "Fluorescence Decay_Decay Pre-Processing:Smoothen Decay", "Fluorescence Decay_Decay Pre-Processing:Extrapolate Decay", "Fluorescence Decay_Decay Pre-Processing:Use Periodicity", "Fluorescence Decay_Decay Pre-Processing:Use Cursors", "Fluorescence Decay_Decay Pre-Processing:Tail Fraction", "Fluorescence Decay_Decay Pre-Processing:Head Fraction", "Fluorescence Decay_Decay Pre-Processing:Additional Points", "Fluorescence Decay_Decay Pre-Processing:Straighten Decay", "Fluorescence Decay_Decay Pre-Processing:Constant Background", "Fluorescence Decay_Decay Pre-Processing:Pixel-Normalize Decay", "Fluorescence Decay_Advanced Analysis:Extract IRF instead of Decay", "Fluorescence Decay_Advanced Analysis:IRF Extraction Options", "Fluorescence Decay_Advanced Analysis:IRF Optimization Options", "Fluorescence Decay_Advanced Analysis:Square Pulse Options", "Fluorescence Decay_Advanced Analysis:IRF Order", "Fluorescence Decay_Advanced Analysis:IRF Time Constants", "Fluorescence Decay_Advanced Analysis:Wavelet Analysis Options", "Fluorescence Decay_Advanced Analysis:Average Lifetime Options", "Fluorescence Decay_Fit Options:Fit Options", "Fluorescence Decay_Fit Options:Use Legacy Fitting Approach", "Fluorescence Decay_Fit Options:Use Data Information Laser Period", "Fluorescence Decay_Fit Parameters:Displayed Fit Parameters", "Fluorescence Decay_Fit Parameters:Fit Parameter Constraints", "Fluorescence Decay_Fit Parameters:Export Tabulated Results", "Fluorescence Decay_Fit Parameters:MLE Baseline Offset Type", "Fluorescence Decay_Fit Parameters:MLE Baseline Offset", "Fluorescence Decay_Fit Parameters:Guess Parameter Names", "Fluorescence Decay_Fit Parameters:Guess Parameter Values", "Fluorescence Decay_Fit Parameters:Guess Parameters Options", "Fluorescence Decay_Styles:Show Last Decay Only", "Fluorescence Decay_Styles:Decay Graph Color Array", "Fluorescence Decay:Decay Graph Active", "Fluorescence Decay Statistics:Min Peak Value", "Fluorescence Decay Statistics:Reject Low Decay Peak Pixels", "Fluorescence Decay Statistics:Reject High Decay Peak Pixels", "Fluorescence Decay Statistics:Max Peak Value", "Time Traces:Use File Timestamp", "Time Traces:Time Step", "Time Traces:Use Intensity Correction File", "Time Traces:Intensity Correction File", "Phasor Plot:Phasor Plot Smoothing Options", "Phasor Plot:Phasor Plot Size", "Phasor Plot:Phasor Plot Graphics Options", "Phasor Plot:Cumulative Phasor Plot", "Phasor Plot:Use Phasor Brightness", "Phasor Plot:Blend Overlay with Phasor Background", "Phasor Plot:Save Phasor Plot", "Phasor Plot:Show References", "Phasor Plot:Phasor Ratio Decay Range", "Phasor Plot:Exponential Fading", "Phasor Plot:Phasor Ratio Reference Colors", "Phasor Plot:Reference Radius", "Phasor Plot:Show Color Map Vertices", "Phasor Plot:Phasor Plot Active", "Phasor Plot:Phasor Ratio Color Map Type", "Phasor Plot:Phasor Ratio Color Map", "Phasor Plot:Phasor Ratio Display Range", "Phasor Plot:Selected Image ROI(s)", "Phasor Plot:All Image ROIs", "Phasor Plot:Selected Phasor Plot ROI(s)", "Phasor Plot:All Phasor Plot ROIs", "Phasor Plot:Phasor Ratio Color-Coded Quantity", "Phasor Plot:Store Phasor Harmonics", "Phasor Plot:Draw Reference Segment", "Phasor Plot:User-Defined Quantity", "Phasor Graph:Phasor Frequency", "Phasor Graph:Phasor Ratio Type", "Phasor Graph:Pixel-level Phasor Computation", "Phasor Graph:Save Phasor Graph", "Phasor Graph:Phasor Graph Active", "Phasor Graph:Phasor SDV Options", "Phasor Calibration:Use Backup Calibration if needed", "Phasor Graph:Define Shortest Lifetime as", "Phasor Calibration:Backup Calibration Type", "Phasor Calibration:Calibration Type", "Phasor Calibration:Calibration Lifetime", "Phasor Calibration:Calibration Map Algorithm", "Single-Exponential Phasor Locus (SEPL):Gate Parameters", "Single-Exponential Phasor Locus (SEPL):User-defined Gate", "Single-Exponential Phasor Locus (SEPL):User-defined IRF", "Single-Exponential Phasor Locus (SEPL):Phasor Parameters", "Single-Exponential Phasor Locus (SEPL):Decay & IRF Parameters", "Single-Exponential Phasor Locus (SEPL):Display Parameters", "Lifetime Analysis:Decay Analysis Parameters", "Lifetime Analysis:Lifetime Map Active", "Plugins:Python Settings", "Miscellaneous:Verbose Mode", "Miscellaneous:Beep after Script", "Miscellaneous:Saved Image File Format", "Miscellaneous:Exported Gate Image Settings", "Miscellaneous:Include Loading in Timing", "Miscellaneous:Verbose Settings Mode", "Miscellaneous:Histogram Options", "Miscellaneous:Beep on Error", "Miscellaneous:# Logical Processors Used", "Miscellaneous:ROI Description Max Characters", "Miscellaneous:Verbose Error Mode", "Miscellaneous:Transparent Mask Color"}
  T53 = typedef "AlliGator Action Engine.lvlib/Alligator Elements Order in Action Stack.ctl" = enum16{"Enqueue 2 AFTER 1", "Enqueue 2 BEFORE 1"}
  T54 = typedef "AlliGator Debug.lvlib/AlliGator Debug Action List.ctl" = enum16{"SS3 Gate Slip Correction", "Test Progress Bar", "Check Reference/IRF Definition", "Fit to Cubic Spline + Sine", "Check SS2 data scrambling", "Remove Image Outliers", "Test Python Plugin", "Edge ROI", "Change Frequency Programmatically", "Open Local Decay Graph Window", "Test Flatfield Correction", "Test Critical Bug"}
  T55 = typedef "AlliGator Action Engine.lvlib/AlliGator Q Element.ctl" = cluster{"AlliGator Q Event":T47, "Data":variant}
  T56 = typedef "AlliGator Action Engine.lvlib/AlliGator Event Category.ctl" = enum16{"GUI", "Files", "FLI Dataset", "FLI Dataset Series", "Image", "Decay", "Intensity Time Trace", "Phasor Plot", "Phasor Graph", "Phasor Ratio", "Calibration", "Decay Fit Parameter Map", "Generic Graph", "DEBUG"}
  T57 = typedef "Notebook.lvlib/Notebook Message Object.ctl" = cluster{"Message":string, "Message Style":T58}
  T58 = typedef "Rich Text Box.lvlib/Text Formatting.ctl" = cluster{"Font":string, "Text Color":T59, "Text Background Color":T59, "Text Style":enum16{"Regular", "Bold", "Italic", "Underline", "Strikeout"}, "Font Size (Points)":dbl, "Text Alignment":i32}
  T59 = typedef "Rich Text Box.lvlib/Text Colors.ctl" = enum16{"Unchanged", "Black", "Blue", "Brown", "Gray", "Green", "Orange", "Pink", "Red", "White"}
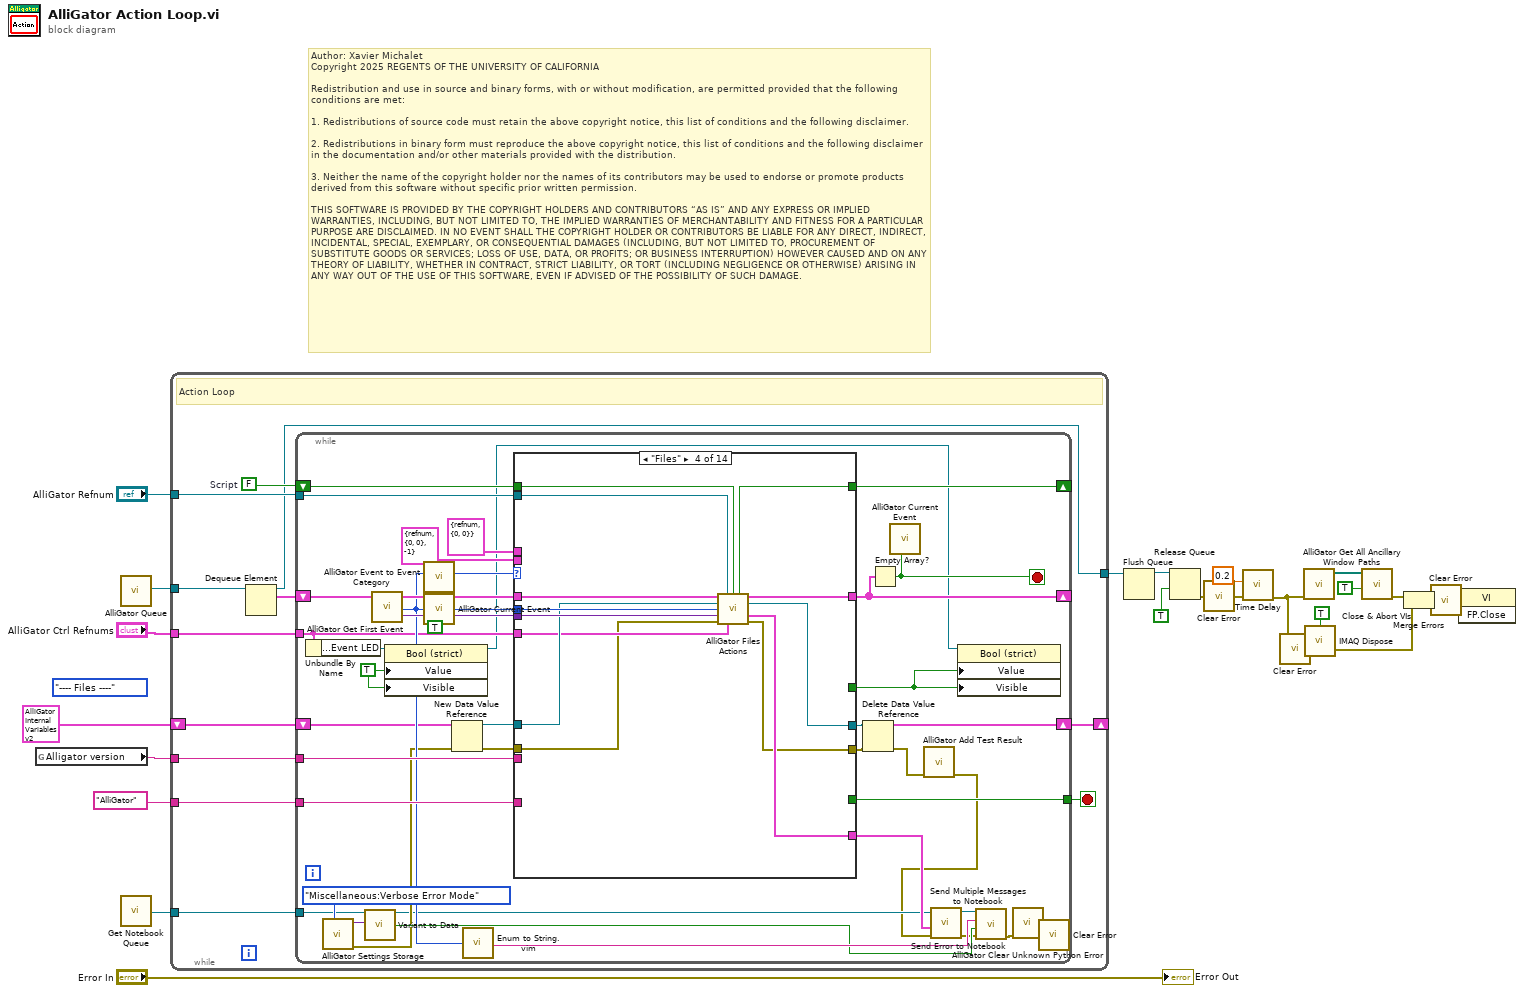
[diagram p0: block diagram]
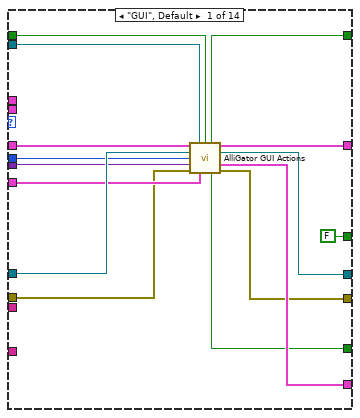
[diagram p2: hidden frame]
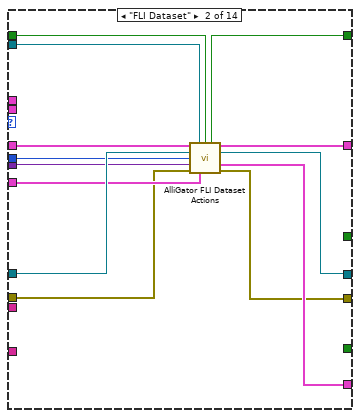
[diagram p3: hidden frame]
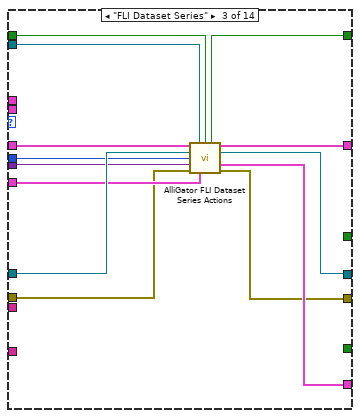
[diagram p4: hidden frame]
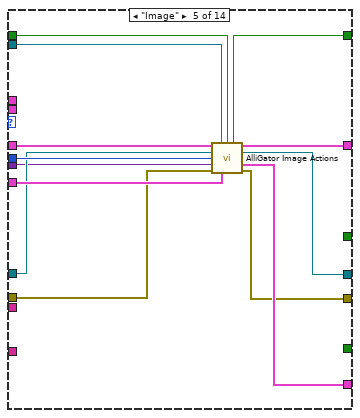
[diagram p5: hidden frame]
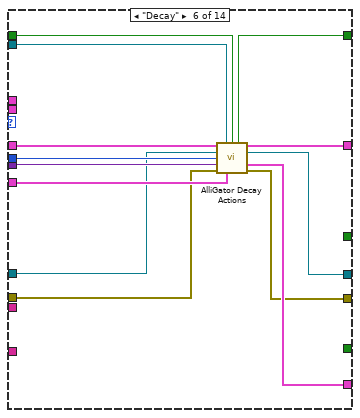
[diagram p6: hidden frame]
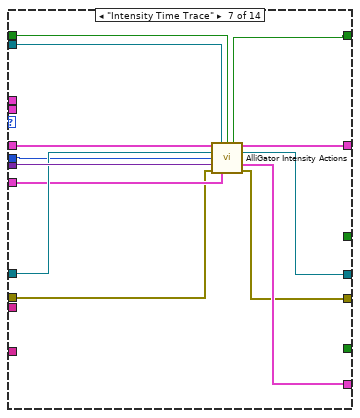
[diagram p7: hidden frame]
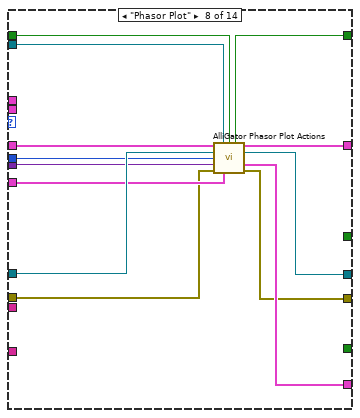
[diagram p8: hidden frame]
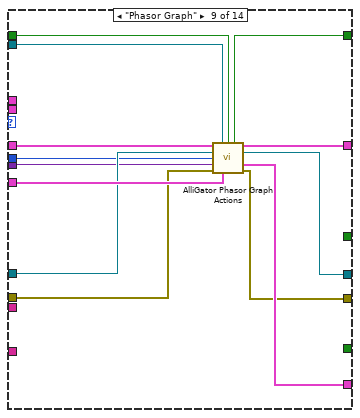
[diagram p9: hidden frame]
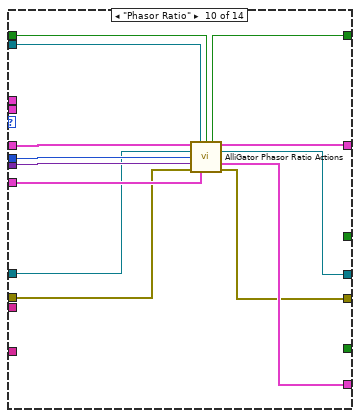
[diagram p10: hidden frame]
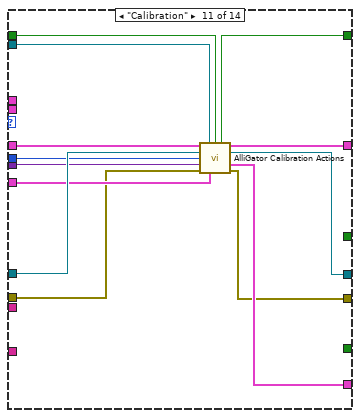
[diagram p11: hidden frame]
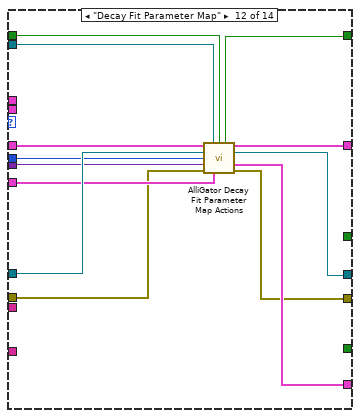
[diagram p12: hidden frame]
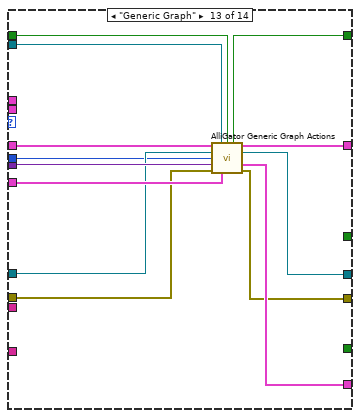
[diagram p13: hidden frame]
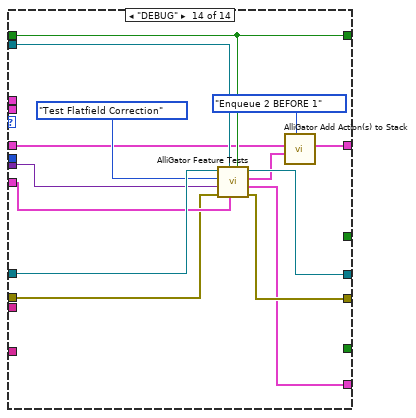
[diagram p14: hidden frame]
diagram:
  (unwired) AlliGator_Q_Event."---- Files ----" ("AlliGator Q Event out")
  # "Author: Xavier Michalet\nCopyright 2025 REGENTS OF THE UNIVERSITY OF CALIFORNIA\n\nRedistribution and use in source and binary forms, with or without modification, are permitted provided that the following conditions are met:\n\n1. Redistributions of source code must retain the above copyright notice, this list of conditions and the following disclaimer.\n\n2. Redistributions in binary form must reproduce the above copyright notice, this list of conditions and the following disclaimer in the documentation and/or other materials provided with the distribution.\n\n3. Neither the name of the copyright holder nor the names of its contributors may be used to endorse or promote products derived from this software without specific prior written permission.\n\nTHIS SOFTWARE IS PROVIDED BY THE COPYRIGHT HOLDERS AND CONTRIBUTORS “AS IS” AND ANY EXPRESS OR IMPLIED WARRANTIES, INCLUDING, BUT NOT LIMITED TO, THE IMPLIED WARRANTIES OF MERCHANTABILITY AND FITNESS FOR A PARTICULAR PURPOSE ARE DISCLAIMED. IN NO EVENT SHALL THE COPYRIGHT HOLDER OR CONTRIBUTORS BE LIABLE FOR ANY DIRECT, INDIRECT, INCIDENTAL, SPECIAL, EXEMPLARY, OR CONSEQUENTIAL DAMAGES (INCLUDING, BUT NOT LIMITED TO, PROCUREMENT OF SUBSTITUTE GOODS OR SERVICES; LOSS OF USE, DATA, OR PROFITS; OR BUSINESS INTERRUPTION) HOWEVER CAUSED AND ON ANY THEORY OF LIABILITY, WHETHER IN CONTRACT, STRICT LIABILITY, OR TORT (INCLUDING NEGLIGENCE OR OTHERWISE) ARISING IN ANY WAY OUT OF THE USE OF THIS SOFTWARE, EVEN IF ADVISED OF THE POSSIBILITY OF SUCH DAMAGE."
  n1 = global read "AlliGator Globals.vi" "Alligator version"() -> (w21:string)
  n2 = call "AlliGator Queue.vi"() -> ("AlliGator Q"=w4:refnum<queue>)  [unwired: 8 in, 1 out]
  n3 = call "Get Notebook Queue.vi"() -> ("Notebook Queue"=w20:refnum<queue>)  [unwired: 9 in]
  n4 = while {
    tunnel: "AlliGator Refnum" -> [w34]
    tunnel: w20 -> [w33]
    shift-right: [w32] -> _
    shift-left: T9 {"Displayed Image"=refnum, "White Light Image"=refnum, "Mask Image"=refnum, "ROI Mask Image"=refnum, "Current Dataset Images 1"={"SGL Image Max"=refnum, "SGL Image Sum"=refnum, "SGL Gate Images"=[], "SGL Image Min"=refnum}, "Background Dataset Images 1"={"SGL Image Max"=refnum, "SGL Image Sum"=refnum, "SGL Gate Images"=[], "SGL Image Min"=refnum}, "Current Dataset Images 2"={"SGL Image Max"=refnum, "SGL Image Sum"=refnum, "SGL Gate Images"=[], "SGL Image Min"=refnum}, "Background Dataset Images 2"={"SGL Image Max"=refnum, "SGL Image Sum"=refnum, "SGL Gate Images"=[], "SGL Image Min"=refnum}, "Current Dataset Arithmetic Images"={"SGL Image Max"=refnum, "SGL Image Sum"=refnum, "SGL Gate Images"=[], "SGL Image Min"=refnum}, "Accumulated Dataset Images 1"={"SGL Image Max"=refnum, "SGL Image Sum"=refnum, "SGL Gate Images"=[], "SGL Image Min"=refnum}, "Accumulated Dataset Images 2"={"SGL Image Max"=refnum, "SGL Image Sum"=refnum, "SGL Gate Images"=[], "SGL Image Min"=refnum}, "Accumulated Dataset Arithmetic Images"={"SGL Image Max"=refnum, "SGL Image Sum"=refnum, "SGL Gate Images"=[], "SGL Image Min"=refnum}, "Phasor Plot Image"=refnum, "Decay Fit Parameter Map Image"=refnum, "Single Data Point Path"=path "", "White Light Image Path"=path "", "Mask Image Path"=path "", "Time-Series Folder"=path "", "[Time-Series Paths]"=[], "Current Dataset"=0, "Single Dataset Type"=enum."HDF5 FLI Dataset", "Current Folder"="", "AlliGator Data Series Type"=enum."HDF5 FLI Dataset Series", "# Datasets"=0, "Dual-Channel Dataset"=FALSE, "Selected Channel Name"="", "Dataset Channel"=enum."G2", "Channel Arithmetic"=enum."None", "Dual-Channel Background Dataset"=FALSE, "Background Channel"=enum."G2", "Dual-Channel Accumulated Dataset"=FALSE, "Start Time"=0.0, "[Time-Series Timestamps]"=[], "[Intensity Corrections]"=[], "Time Series Script"=FALSE, "Type of Displayed Image"=enum."Sum of All Gates", "Gate Image Slide"=0, "# Gates"=0, "ROIs"=[], "ROI Decay"={"t Array"=[], "I Array"=[]}, "Valid Decay"=FALSE, "Decay  Metadata"={"ROI Descriptor"={"Global Rectangle"=[], "Contours"=[]}, "ROI Center"={"X"=0, "Y"=0}, "Decay Background Subtraction Info"={"Laser Period"=0.0, "Gate Duration"=0.0, "Baseline Subtraction Method"=enum."Mean", "Background Definition Range"={"Min Gate"=0.0, "Max Gate"=0.0}, "Total Intensity w/o Bkgd Subtraction"=0.0, "Bkgd-subtracted Intensity (exp)"=0.0, "# Data Points"=0, "Background/Gate"=0.0, "Fitted Lifetime"=0.0, "Bkgd-subtracted Intensity (theo)"=0.0}, "Decay Reverted"=FALSE, "Decay Smoothened"=FALSE, "Decay Straightened"=FALSE, "Fitted Tau (Decay Straightening)"=0.0, "Decay Shift Parameters"={"Type"=enum."Default", "Shift"=0.0, "Threshold"=0.0, "Rotate"=FALSE}, "Decay Shifted"=FALSE, "Decay Extrapolated"=FALSE, "Decay Extrapolation Parameters"={"Additional Points"=0, "Head Fraction"=0.0, "Fitted Tau"=0.0, "Use Periodicity"=FALSE, "Use Cursors"=FALSE, "Tail Fraction"=0.0}, "Decay Normalized"=FALSE, "Fold Decay"=FALSE, "# Folds"=1}, "Reference Decay Plot Name"="", "Reference Decay"={"t Array"=[], "I Array"=[]}, "Decay Shift Plot"={"Time Stamps"=[], "Decay Shifts"=[]}, "[Decays Max Values]"=[], "[Decays Min Values]"=[], "Calibration Phasor"={"m"=0.0, "phi"=0.0, "Phasor Frequency"=0.0, "Reference Lifetime"=0.0}, "Calibration Phasor Series"={"m Array"=[], "phi Array"=[], "Phasor Frequency"=0.0, "Calibration Lifetime"=0.0}, "Phasor Calibration Map"={"Phasor Frequency"=80000000.0, "Calibration Lifetime"=1e-09, "ROI Centers"=[], "ROI Descriptors"=[], "Map Resolution X"=0, "Map Resolution Y"=0, "z Array"=[]}, "Calibration Map MD5 Digest"="", "Last Raw Phasor"={"g"=0.0, "s"=0.0}, "Last Calibrated Phasor"={"g"=0.0, "s"=0.0}, "Last Calibrated Phasor SDV"={"g"=0.0, "s"=0.0}, "Phasor Graph:Phasor Plot"={"g Array"=[], "s Array"=[]}, "Phasor Graph:Phasor SDV Plot"={"g Array"=[], "s Array"=[]}, "[Phasor Graph:Raw Phasor Plots]"=[], "Phasor Plot locked to Ref 1"=-1, "[Phasor Plot(s) locked to Ref 1]"=[], "[Phasor Plot(s) locked to Ref 2]"=[], "[Pixel Phasors]"=[], "[[Sum Image]]"=[], "[[CSG Phasors]]"=[], "[[Valid Pixel?]]"=[], "I/m/phi Dataset"={"I/m/phi Dataset?"=FALSE, "Base Frequency"=0.0, "Harmonic Orders"=[]}, "Multi Phasor Plot Data"={"Base Frequency"=0.0, "# Harmonics"=0, "Harmonic Orders"=[], "Phasor Plot Settings Checksum"=0, "Phasor Harmonic Data Array"=[]}, "Decay Fit Options & Parameters"={"SYNC Period"=0.0, "Fit Options"={"Show Fit Residuals"=FALSE, "Fit Model"=enum."1-Exponential", "Residual Type"=enum."Standard", "Max Decay Percentile"=0.0, "Min Decay Percentile"=0.0, "Show Full Decay"=FALSE, "Weights"=enum."Unweighted", "Fitting Method"=enum."Least Square", "Compute Parameter Uncertainties"=FALSE, "Periodic Boundaries"=FALSE, "Model Calculation"=enum."Simulation", "Period"=0.0, "Termination Criteria"={"Max Iterations"=0, "Max Function Calls"=0, "Max Time"=0.0, "Function Tolerance"=0.0, "Parameter Tolerance"=0.0, "Gradient Tolerance"=0.0, "Min Lambda"=0.0, "Max Lambda"=0.0, "Initial Tick Count"=0}, "Offset Resolution"=0.0, "Use Local IRF"=FALSE, "Fitting Algorithm"=enum."Levenberg-Marquardt"}, "Fit Parameter Constraints"=[], "MLE Baseline Offset"=0.0, "MLE Baseline Offset Type"=enum."Absolute"}, "Fit Options: Decay Preprocessing Parameters"={"Background Subtraction"=FALSE, "Straighten Decay"=FALSE, "Reverse Gates"=FALSE, "1-Normalized Decay"=FALSE, "Smoothen Decay"=FALSE, "Smoothing Parameter"=0.0, "Shift Decay"=FALSE, "Decay Shift Parameters"={"Type"=enum."Default", "Shift"=0.0, "Threshold"=0.0, "Rotate"=FALSE}, "Extrapolate Decay"=FALSE, "Additional Points"=0, "Head Fraction"=0.0, "Pixel-Normalize Decay"=FALSE, "Use Periodicity"=FALSE, "Use Cursors"=FALSE, "Tail Fraction"=0.0, "Use Decay Pre-Processing"=TRUE, "Fold Decay"=FALSE, "# Folds"=1, "[0-1]-Normalized Decay"=FALSE}, "Fit Options: Reference Decay"={"t Array"=[], "I Array"=[]}, "Is Full Image Parameters Map"=FALSE, "Is Single-Pixels Parameters Map"=FALSE, "NLSF Parameters Map X Resolution"=0, "NLSF Parameters Map Y Resolution"=0, "[Single Decay Fit Parameters]"=[], "Fit Model"=enum."1-Exponential", "[[Multiple Decays Fit Parameters]]"=[], "[[Multiple Decays Fit Parameter SDVs]]"=[], "[[IRFs]]"=[], "IRF Array Time Axis"=[], "Decay Array Time Axis"=[], "[Decay Fit Parameter Names]"=[], "[[Phasor Ratios]]"=[], "[[Average Lifetimes]]"=[], "Amplitude Weighted Average Lifetime"=FALSE, "[Decay Sum]"=[], "Parameter Maps"=[], "[[User-defined Quantities]]"=[], "User-defined Quantity"=""} ("AlliGator Internal Variables") -> [w26]
    tunnel: w21 -> [w31]
    tunnel: "AlliGator" ("Sender") -> [w29]
    tunnel: "AlliGator Ctrl Refnums" -> [w28]
    tunnel: w4 -> [w24]
    tunnel: [w25] -> w8
    stop <- w27 stop-if-true
    w30 = FALSE  # Script
    # "Action Loop"
    n5 = Dequeue Element(queue=w24) -> (queue out=w25:refnum<queue>, element=w35:T55[])  [unwired: 2 in, 2 out]
    n6 = while {
      tunnel: [w40] -> w27
      shift-right: [w75] -> _
      shift-left: w35 -> [w70]
      tunnel: w34 -> [w72]
      tunnel: w33 -> [w37]
      shift-right: [w55] -> w32
      shift-left: w26 -> [w58]
      tunnel: w31 -> [w74]
      shift-right: [w54] -> _
      shift-left: w30 -> [w73]
      tunnel: w29 -> [w71]
      tunnel: w28 -> [w53]
      stop <- w62 stop-if-true
      w44 = TRUE ("Value")
      n7 = Unbundle By Name(w53) -> ("Other AlliGator Ctrl Refnums.Event LED"=w52:refnum<vi>)
      n8 = call "AlliGator Settings Storage.vi"("AlliGator Settings List"=AlliGator_Settings_List."Miscellaneous:Verbose Error Mode") -> ("Error Out"=w48:errorcluster, "Variant Data out"=w67:variant)  [unwired: 9 in]
      n9 = call-poly "Variant to Data.vi"("Variant"=w67) -> ("Value"=w50:bool)  [unwired: 8 in]
      n10 = call "AlliGator Get First Event.vi"("AlliGator Q Elements"=w70) -> ("Data"=w69:variant, "AlliGator Q Event"=w61:T47, "AlliGator Q Elements"=w76:T55[])  [unwired: 2 in]
      n11 = property class="Bool (strict)"(reference=w52, "Value"=w44, "Visible"=w44) -> (reference out=w41:refnum<vi>)  [unwired: 1 in, 1 out]
      n12 = call "AlliGator Event to Event Category.vi"("AlliGator Q Event"=w61) -> ("Event Category"=w64:T56)  [unwired: 8 in]
      n13 = call "AlliGator Current Event.vi"("AlliGator Q Event in"=w61, "Get(F)/Set"=TRUE) -> ("AlliGator Q Event out"=w59:T47)  [unwired: 7 in]
      n14 = New Data Value Reference(data value=w58, error in=w48) -> (data value reference=w57:refnum<data-value>, error out=w47:errorcluster)
      n15 = call "Enum to String.vim"("Enum"=w61) -> ("String"=w51:string)
      n16 = case shown="\"Files\"" w64 {
        tunnel: [FALSE ("Quit?") _ _ _ _ _ _ _ _ _ _ _ _ _] -> w45
        tunnel: w76 -> [w91 w104 w117 w130 w143 w150 w169 w180 w195 w202 w218 w234 w247 w252]
        tunnel: [w90 w103 w116 w129 w142 w149 w168 w179 w194 w200 w221 w233 w246 w250] -> w75
        tunnel: w74 -> [_ _ _ _ _ _ _ _ _ _ _ _ _ _]
        tunnel: w73 -> [w87 w100 w113 w123 w136 w156 w157 w174 w193 w208 w213 w223 w239 w255]
        tunnel: w72 -> [w85 w98 w111 w128 w141 w155 w167 w177 w187 w203 w219 w230 w245 w261]
        tunnel: w71 -> [_ _ _ _ _ _ _ _ _ _ _ _ _ _]
        tunnel: w69 -> [w83 w96 w109 w127 w135 w153 w166 w175 w189 w204 w215 w228 w244 w257]
        tunnel: T51 {"Multiplot XY Graph"=refnum, "Mouse Coordinates"={"Horizontal"=0, "Vertical"=0}, "Plot Index"=-1} ("Selected Plot Info") -> [_ _ _ _ _ _ _ _ _ _ _ _ _ _]
        tunnel: w53 -> [w82 w95 w108 w122 w140 w154 w163 w181 w192 w205 w214 w227 w243 w256]
        tunnel: T48 {"Multiplot XY Graph"=refnum, "Mouse Coordinates"={"Horizontal"=0, "Vertical"=0}} ("Mouse Click Event Data") -> [_ _ _ _ _ _ _ _ _ _ _ _ _ _]
        tunnel: w59 -> [w84 w97 w110 w126 w139 w152 w162 w176 w188 w206 w216 w229 w240 _]
        tunnel: w57 -> [w89 w102 w115 w125 w138 w147 w165 w182 w191 w201 w220 w232 w242 w260]
        tunnel: [w88 w101 w114 w124 w137 w148 w164 w178 w190 w199 w217 w231 w241 w259] -> w56
        tunnel: [w86 w99 w112 w121 w134 w151 w158 w170 w186 w207 w209 w222 w235 w255] -> w54
        tunnel: [w81 w94 w107 w120 w133 w146 w161 w173 w185 w198 w212 w226 w238 w248] -> w38
        tunnel: w47 -> [w80 w93 w106 w119 w132 w145 w160 w172 w184 w197 w211 w225 w237 w254]
        tunnel: [w79 w92 w105 w118 w131 w144 w159 w171 w183 w196 w210 w224 w236 w253] -> w46
        tunnel: [w78 _ _ _ _ _ _ _ _ _ _ _ _ _] -> w40
        frame "GUI", Default {
          n17 = call "AlliGator GUI Actions.vi"("AlliGator Q Elements in"=w91, "VI in"=w85, "Script"=w87, "AlliGator IV DVR"=w89, "AlliGator Q Event in"=w84, "Data"=w83, "error in (no error)"=w80, "AlliGator Ctrl Refnums"=w82) -> ("Script?"=w86:bool, "AlliGator Q Elements out"=w90:T55[], "AlliGator IV DVR"=w88:refnum<data-value>, "[Notebook Message]"=w81:T57[], "Quit?"=w78:bool, "error out"=w79:errorcluster)  [unwired: 2 in]
        }
        frame "FLI Dataset" {
          n18 = call "AlliGator FLI Dataset Actions.vi"("AlliGator Q Elements"=w104, "VI in"=w98, "Script in"=w100, "AlliGator IV DVR in"=w102, "AlliGator Q Event in"=w97, "Data"=w96, "error in (no error)"=w93, "AlliGator Ctrl Refnums"=w95) -> ("Script out"=w99:bool, "Alligator Queue Elements"=w103:T55[], "AlliGator IV DVR out"=w101:refnum<data-value>, "[Notebook Message]"=w94:T57[], "error out"=w92:errorcluster)  [unwired: 3 in]
        }
        frame "FLI Dataset Series" {
          n19 = call "AlliGator FLI Dataset Series Actions.vi"("AlliGator Q Elements"=w117, "VI in"=w111, "Script in"=w113, "AlliGator IV DVR in"=w115, "AlliGator Q Event in"=w110, "Data"=w109, "error in (no error)"=w106, "AlliGator Ctrl Refnums"=w108) -> ("Script out"=w112:bool, "Alligator Queue Elements"=w116:T55[], "AlliGator IV DVR out"=w114:refnum<data-value>, "[Notebook Message]"=w107:T57[], "error out"=w105:errorcluster)  [unwired: 3 in]
        }
        frame "Files" {
          n20 = call "AlliGator Files Actions.vi"("AlliGator Q Elements in"=w130, "VI in"=w128, "Script in"=w123, "AlliGator IV DVR"=w125, "AlliGator Q Event in"=w126, "Data"=w127, "error in (no error)"=w119, "AlliGator Ctrl Refnums"=w122) -> ("Script out"=w121:bool, "AlliGator Q Elements out"=w129:T55[], "AlliGator IV DVR"=w124:refnum<data-value>, "[Notebook Message]"=w120:T57[], "error out"=w118:errorcluster)  [unwired: 3 in]
        }
        frame "Image" {
          n21 = call "AlliGator Image Actions.vi"("AlliGator Q Elements"=w143, "VI in"=w141, "Script in"=w136, "AlliGator IV DVR in"=w138, "AlliGator Q Event in"=w139, "Data"=w135, "error in (no error)"=w132, "AlliGator Ctrl Refnums"=w140) -> ("Script out"=w134:bool, "Alligator Queue Elements"=w142:T55[], "AlliGator IV DVR out"=w137:refnum<data-value>, "[Notebook Message]"=w133:T57[], "error out"=w131:errorcluster)  [unwired: 3 in]
        }
        frame "Decay" {
          n22 = call "AlliGator Decay Actions.vi"("AlliGator Q Elements in"=w150, "VI in"=w155, "Script in"=w156, "AlliGator IV DVR in"=w147, "AlliGator Q Event in"=w152, "Data"=w153, "error in (no error)"=w145, "AlliGator Ctrl Refnums"=w154) -> ("Script off"=w151:bool, "AlliGator Q Elements out"=w149:T55[], "AlliGator IV DVR out"=w148:refnum<data-value>, "[Notebook Message]"=w146:T57[], "error out"=w144:errorcluster)  [unwired: 3 in]
        }
        frame "Intensity Time Trace" {
          n23 = call "AlliGator Intensity Actions.vi"("AlliGator Q Elements in"=w169, "VI in"=w167, "Script in"=w157, "AlliGator IV DVR in"=w165, "AlliGator Q Event in"=w162, "Data"=w166, "error in (no error)"=w160, "AlliGator Ctrl Refnums"=w163) -> ("Script out"=w158:bool, "AlliGator Q Elements out"=w168:T55[], "AlliGator IV DVR out"=w164:refnum<data-value>, "[Notebook Message]"=w161:T57[], "error out"=w159:errorcluster)  [unwired: 3 in]
        }
        frame "Phasor Plot" {
          n24 = call "AlliGator Phasor Plot Actions.vi"("AlliGator Q Elements in"=w180, "VI in"=w177, "Script in"=w174, "data value reference in"=w182, "AlliGator Q Event in"=w176, "Data"=w175, "error in (no error)"=w172, "AlliGator Ctrl Refnums"=w181) -> ("Script out"=w170:bool, "AlliGator Q Elements out"=w179:T55[], "Data Value Reference out"=w178:refnum<data-value>, "[Notebook Message]"=w173:T57[], "error out"=w171:errorcluster)  [unwired: 3 in]
        }
        frame "Phasor Graph" {
          n25 = call "AlliGator Phasor Graph Actions.vi"("AlliGator Q Elements in"=w195, "VI in"=w187, "Script in"=w193, "Data Value Reference in"=w191, "AlliGator Q Event in"=w188, "Data"=w189, "error in (no error)"=w184, "AlliGator Ctrl Refnums"=w192) -> ("Script out"=w186:bool, "AlliGator Q Elements out"=w194:T55[], "Data Value Reference out"=w190:refnum<data-value>, "[Notebook Message]"=w185:T57[], "error out"=w183:errorcluster)  [unwired: 3 in]
        }
        frame "Phasor Ratio" {
          n26 = call "AlliGator Phasor Ratio Actions.vi"("AlliGator Q Elements in"=w202, "VI in"=w203, "Script in"=w208, "data value reference in"=w201, "AlliGator Q Event in"=w206, "Data"=w204, "error in (no error)"=w197, "AlliGator Ctrl Refnums"=w205) -> ("Script out"=w207:bool, "AlliGator Q Elements out"=w200:T55[], "Data Value Reference out"=w199:refnum<data-value>, "[Notebook Message]"=w198:T57[], "error out"=w196:errorcluster)  [unwired: 3 in]
        }
        frame "Calibration" {
          n27 = call "AlliGator Calibration Actions.vi"("AlliGator Q Elements"=w218, "VI in"=w219, "Script in"=w213, "data value reference"=w220, "AlliGator Q Event in"=w216, "Data"=w215, "error in (no error)"=w211, "AlliGator Ctrl Refnums"=w214) -> ("Script out"=w209:bool, "Alligator Queue Element 1 (+ 2)"=w221:T55[], "AlliGator IV DVR"=w217:refnum<data-value>, "[Notebook Message]"=w212:T57[], "error out"=w210:errorcluster)  [unwired: 3 in]
        }
        frame "Decay Fit Parameter Map" {
          n28 = call "AlliGator Decay Fit Parameter Map Actions.vi"("AlliGator Q Elements in"=w234, "VI in"=w230, "Script in"=w223, "data value reference"=w232, "AlliGator Q Event in"=w229, "Data"=w228, "error in (no error)"=w225, "AlliGator Ctrl Refnums"=w227) -> ("Script out"=w222:bool, "AlliGator Q Elements out"=w233:T55[], "Data Value Reference out"=w231:refnum<data-value>, "[Notebook Message]"=w226:T57[], "error out"=w224:errorcluster)  [unwired: 3 in]
        }
        frame "Generic Graph" {
          n29 = call "AlliGator Generic Graph Actions.vi"("AlliGator Q Elements in"=w247, "VI in"=w245, "Script"=w239, "data value reference in"=w242, "AlliGator Q Event in"=w240, "Data"=w244, "error in (no error)"=w237, "AlliGator Ctrl Refnums"=w243) -> ("Script out"=w235:bool, "AlliGator Q Elements out"=w246:T55[], "Data Value Reference out"=w241:refnum<data-value>, "[Notebook Message]"=w238:T57[], "error out"=w236:errorcluster)  [unwired: 3 in]
        }
        frame "DEBUG" {
          n30 = call "AlliGator Feature Tests.vi"("Script"=w255, "AlliGator Ctrl Refnums"=w256, "VI in"=w261, "Error In"=w254, "Data"=w257, "Debug Action List"=AlliGator_Debug_Action_List."Test Flatfield Correction", "data value reference"=w260) -> ("Error Out"=w253:errorcluster, "[Notebook Message]"=w248:T57[], "AlliGator Action"=w251:T55[], "Data Value Reference out"=w259:refnum<data-value>)  [unwired: 1 in]
          n31 = call-poly "AlliGator Add Action(s) to Stack.vi"("Elements Order in Action Stack (Default: 2 BEFORE 1)"=Alligator_Elements_Order_in_Action_Stack."Enqueue 2 BEFORE 1", "Alligator Queue Element 2"=w251, "Alligator Queue Element 1"=w252) -> ("Alligator Queue Element 1 (+ 2)"=w250:T55[])  [unwired: 7 in, 1 out]
        }
      }
      n32 = Delete Data Value Reference(data value reference=w56, error in=w46) -> (data value=w55:T9, error out=w39:errorcluster)
      n33 = Empty Array?(array=w75) -> (empty?=w62:bool)
      n34 = call "AlliGator Current Event.vi"("Get(F)/Set"=w62) -> ()  [unwired: 8 in, 1 out]
      n35 = call "AlliGator Add Test Result.vi"("error in (no error)"=w39) -> ("error out"=w36:errorcluster)  [unwired: 10 in]
      n36 = call "Send Multiple Messages to Notebook.vi"("Error In"=w36, "[Notebook Message]"=w38, "Notebook Queue"=w37) -> ("Error Out"=w42:errorcluster, "Notebook Queue"=w43:refnum<queue>)  [unwired: 5 in]
      n37 = property class="Bool (strict)"(reference=w41, "Value"=w45, "Visible"=w45) -> ()  [unwired: 1 in, 2 out]
      n38 = call "Send Error to Notebook.vi"("error in (no error)"=w42, "Verbose Error Messages (T)"=w50, "State Machine Case Error Source"=w51, "Notebook Q"=w43) -> ("Error Out"=w65:errorcluster)  [unwired: 7 in]
      n39 = call "AlliGator Clear Unknown Python Error.vi"("error in (no error)"=w65) -> ("error out"=w49:errorcluster)  [unwired: 10 in]
      n40 = call "Clear Error.vi"("Error In"=w49) -> ()  [unwired: 8 in, 1 out]
    }
  }
  n41 = Flush Queue(queue=w8) -> (queue out=w7:refnum<queue>)  [unwired: 1 in, 2 out]
  n42 = Release Queue(queue=w7, force destroy? (F)=TRUE) -> (error out=w5:errorcluster)  [unwired: 1 in, 2 out]
  n43 = call "Clear Error.vi"("Error In"=w5) -> ("no Error Out"=w3:errorcluster)  [unwired: 8 in]
  n44 = call "Time Delay"("error in (no error)"=w3, "Delay Time (s)"=0.2 ("milliseconds to wait")) -> ("error out"=w2:errorcluster)  [unwired: 9 in]
  n45 = call "Clear Error.vi"("Error In"=w2) -> ("no Error Out"=w9:errorcluster)  [unwired: 8 in]
  n46 = call "AlliGator Get All Ancillary Window Paths.vi"("Error In"=w2) -> ("AlliGator Window Paths"=w17:path[])  [unwired: 9 in, 1 out]
  n47 = call "IMAQ Dispose"("All Images? (No)"=TRUE, "error in (no error)"=w9) -> ("error out"=w13:errorcluster)  [unwired: 4 in]
  n48 = call "Close & Abort VIs.vi"("Abort (T)"=TRUE, "VI Paths"=w17) -> ("Error Out"=w16:errorcluster)  [unwired: 9 in]
  n49 = Merge Errors(w16, w13) -> (w14:errorcluster)
  n50 = call "Clear Error.vi"("Error In"=w14) -> ("no Error Out"=w12:errorcluster)  [unwired: 8 in]
  n51 = invoke class="VI" method="FP.Close"(error in=w12) -> ()  [unwired: 2 in, 3 out]
  "Error Out" <- "Error In"
